vi "VMI_acquire_subV_Arrays.vi"(0 "Big_image Array":i16[][][](array[numeric]), 2 "Queue Array":T7[](array[typedef]), 4 "IMAQ In":T4, 5 "error in (no error)":errorcluster, 7 "Types to acquire in":bool[](array[boolean]), 9 "Collection Information":T1[](array[typedef]), 10 "Peak Find Settings":T6, 11 "Session Out":T3, 13 "Ref Cluster 1":T2) -> (12 "Points per image":i32[](array[numeric]), 14 "IMAQ out":T4, 15 "Histogram_array":i32[][](array[numeric]), 16 "Signal Background":cluster{"X":sgl, "Y":sgl}[](array[cluster]), 17 "Background":cluster{"X":sgl, "Y":sgl}[](array[cluster]), 18 "Background 2":cluster{"X":sgl, "Y":sgl}[](array[cluster]), 19 "error out":errorcluster)   [LabVIEW 2018]
uses:
  <vilib>/vision/Image Controls.llb/IMAQ Image.ctl
  <vilib>/userdefined/High Color/IMAQdx.ctl
  Type defs/Ref_cluster.ctl
  Type defs/FileAcq_v1_Ctrl.ctl
panel:
  out "Graph X":i32[](array[numeric])
  in  "Back2_Points_Image":i32[](array[numeric])
  in  "Back1_Points_Image":i32[](array[numeric])
  in  "Signal_Points_Image":i32[](array[numeric])
  in  "Types to acquire settings":T5(array[cluster])
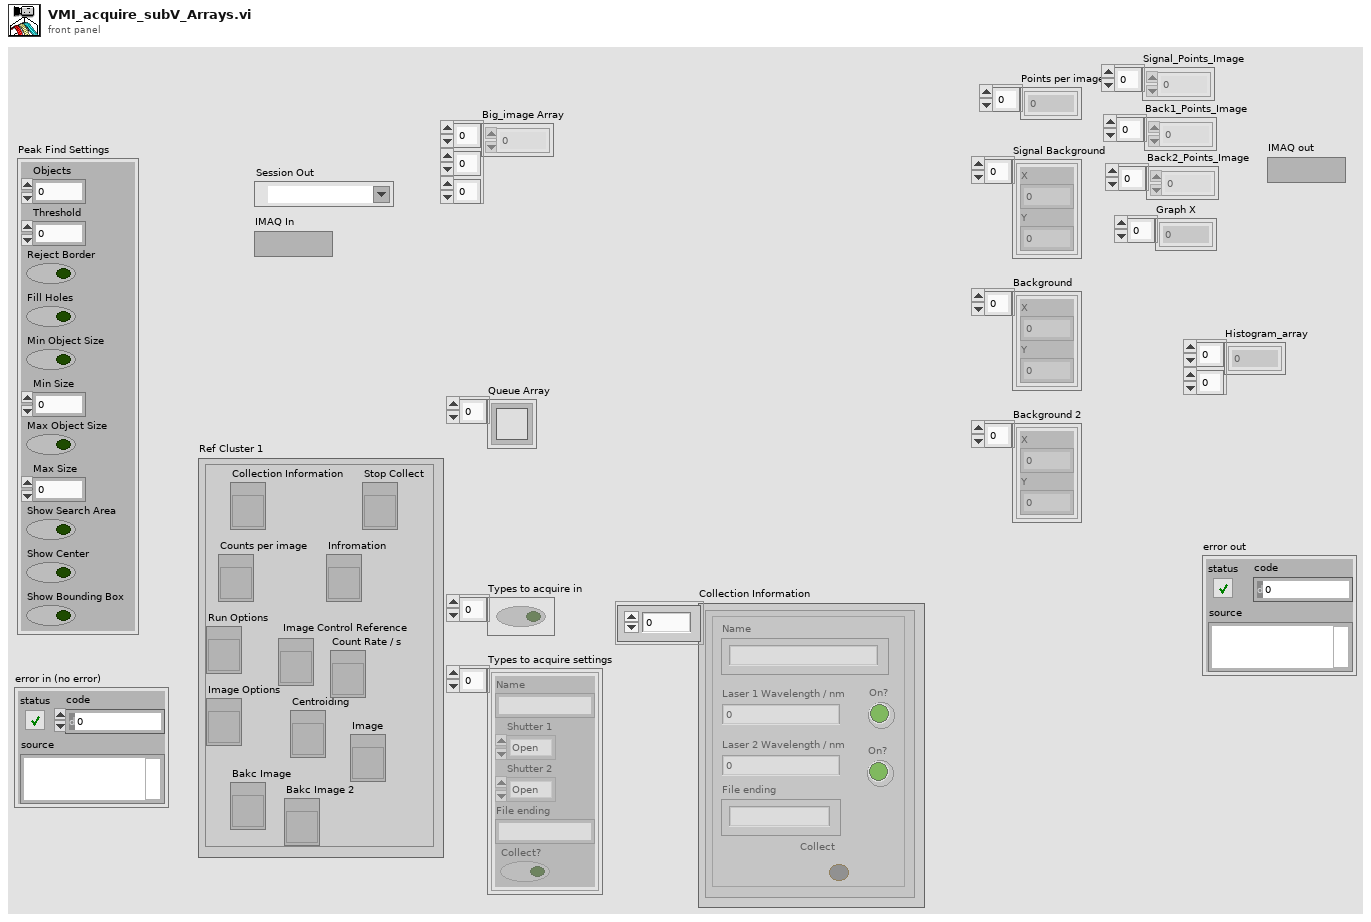
[diagram p1: front panel]
types:
  T1 = typedef "FileAcq_v1_Ctrl.ctl" = cluster{"Type":string, "LaserWave1":dbl, "Shutter1":bool, "LaserWave2":dbl, "Shutter2":bool, "FileEnd":string, "Collect":bool}
  T2 = typedef "Ref_cluster.ctl" = cluster{"Stop Collect ":refnum<vi>, "Collection Information ":refnum<vi>, "Infromation":refnum<vi>, "Counts per image":refnum<vi>, " Image Control Reference ":refnum<vi>, "Run Options":refnum<vi>, "Image Options":refnum<vi>, "Centroiding":refnum<vi>, "Image":refnum<vi>, "Bakc Image":refnum<vi>, "Bakc Image 2":refnum<vi>, "Count Rate / s":refnum<vi>}
  T3 = typedef "IMAQdx.ctl" = refnum<k21>
  T4 = typedef "IMAQ Image.ctl" = refnum<image>
  T5 = cluster{"Name":string, "Shutter 1":enum16{"Open", "Closed"}, "Shutter 2":enum16{"Open", "Closed"}, "File ending":string, "Collect?":bool}[]
  T6 = cluster{"Objects":u16, "Threshold":i32, "Reject Border":bool, "Fill Holes":bool, "Min Object Size":bool, "Min Size":i32, "Max Object Size":bool, "Max Size":i32, "Show Search Area":bool, "Show Center":bool, "Show Bounding Box":bool}
  T7 = typedef "Queue RefNum" = refnum<k1>
  T8 = typedef "Image Type" = u32
  T9 = cluster{"Total Time / ms":dbl, "Image Total Collection Time":dbl, "Image Loop time / ms":dbl, "Peak Total Find Time":dbl, "Peak Find Time / ms":dbl, "Camera Rate / Hz":dbl, "Total Number of Loops":dbl, "Current Loop Number":dbl, "Number of Image Loops":dbl, "Run Mode":dbl}
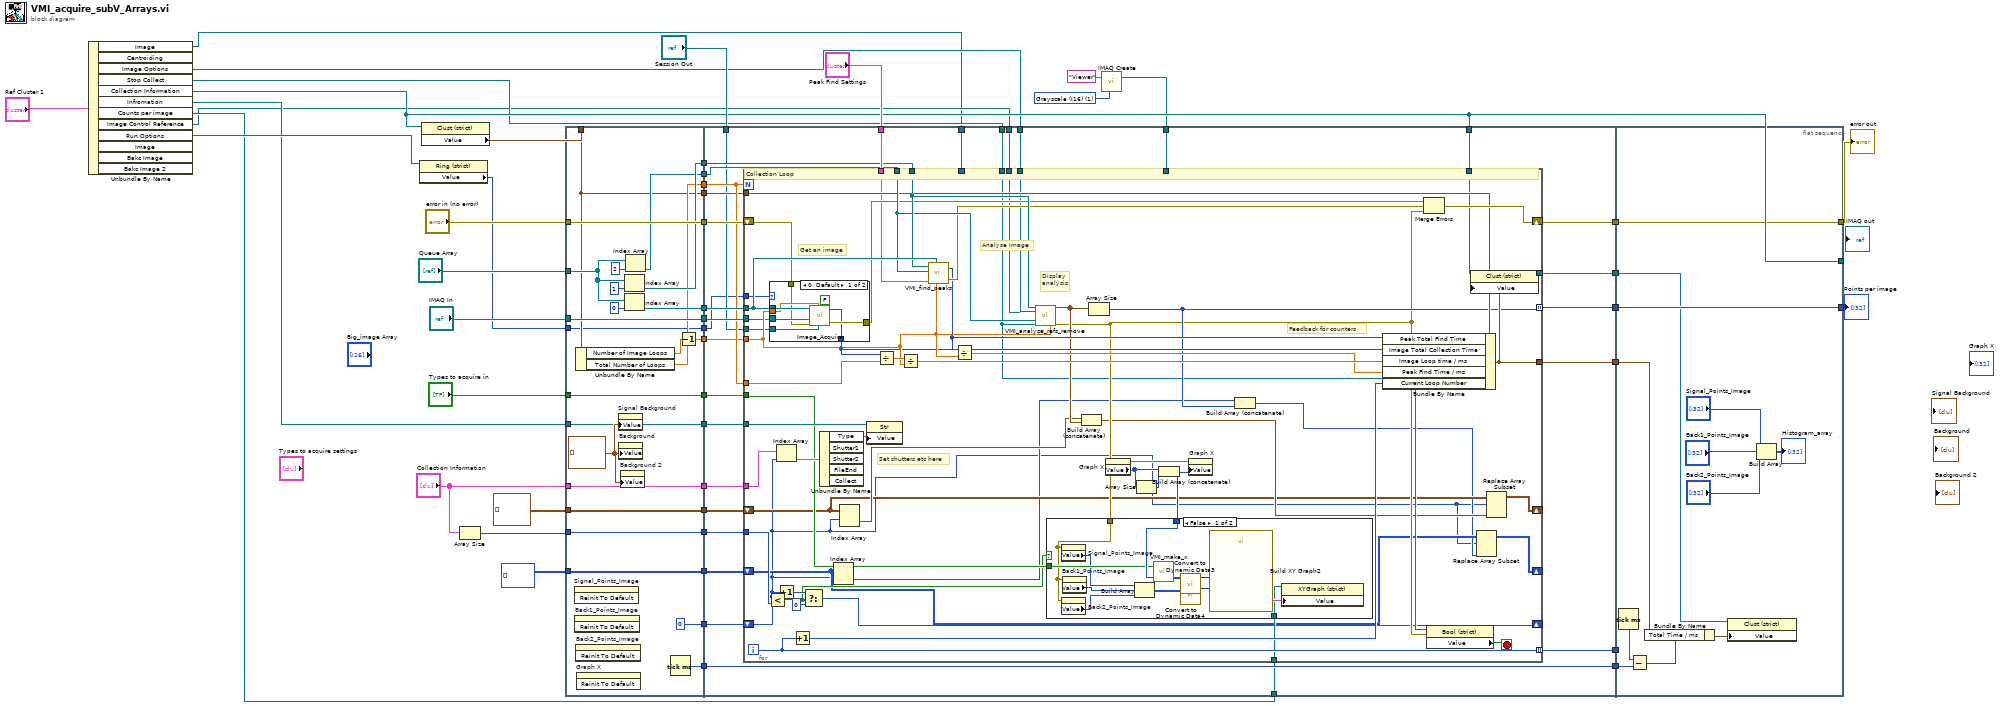
[diagram p0: block diagram]
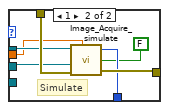
[diagram p2: hidden frame]
diagram:
  w9 = T8 1 items=["Grayscale (U8)", "Grayscale (I16)", "Grayscale (SGL)", "Complex (CSG)", "RGB (U32)", "HSL (U32)", "RGB (U64)", "Grayscale (U16)"] ("Image Type")
  n1 = Unbundle By Name("Ref Cluster 1") -> ("Image"=w12:refnum<vi>, "Image Options"=w13:refnum<vi>, "Stop Collect"=w17:refnum<vi>, "Collection Information"=w19:refnum<vi>, "Infromation"=w15:refnum<vi>, "Counts per image"=w18:refnum<vi>, "Image Control Reference"=w14:refnum<vi>, "Run Options"=w22:refnum<vi>)  [unwired: 4 out]
  n2 = property class="Ring (strict)"(reference=w22) -> ("Value"=w20:u16)  [unwired: 1 in, 2 out]
  n3 = property class="Clust (strict)"(reference=w19) -> ("Value"=w25:T9)  [unwired: 1 in, 2 out]
  n4 = Array Size(array="Collection Information") -> (size(s)=w4:i32)
  n5 = flat-sequence {
    tunnel: "error in (no error)" -> [w70]
    tunnel: "Collection Information" -> [w71]
    tunnel: "IMAQ In" -> [w72]
    tunnel: [w65] -> w49
    tunnel: [w72] -> w48
    tunnel: [w71] -> w47
    tunnel: [w70] -> w46
    tunnel: [w57] -> w45
    tunnel: [w58] -> w44
    tunnel: [w69] -> w43
    tunnel: [0] -> w42
    tunnel: [w68] -> w41
    tunnel: "Types to acquire in" -> [w68]
    tunnel: [w56] -> w40
    tunnel: "Queue Array" -> [w61]
    tunnel: [w63] -> w39
    tunnel: [w60] -> w38
    tunnel: w25 -> [w56]
    tunnel: [w54] -> w21
    tunnel: w20 -> [w54]
    tunnel: [w53] -> w16
    tunnel: w15 -> [w53]
    tunnel: cluster{"X":sgl, "Y":sgl}[][] [] -> [w52]
    tunnel: [w52] -> w6
    tunnel: w4 -> [w51]
    tunnel: [w51] -> w3
    tunnel: [w50] -> w2
    tunnel: i32[][] [] ("Histogram_array 2") -> [w50]
    tunnel: [w102] -> w37
    tunnel: [w99] -> w36
    tunnel: [w98] -> w35
    tunnel: w49 -> [w103]
    tunnel: w48 -> [w101]
    tunnel: w47 -> [w100]
    tunnel: w46 -> [w97]
    tunnel: w45 -> [w96]
    tunnel: w44 -> [w95]
    tunnel: [w94] -> w34
    tunnel: w43 -> [w94]
    tunnel: w42 -> [w93]
    tunnel: w41 -> [w85]
    tunnel: w40 -> [w92]
    tunnel: [w91] -> w33
    tunnel: "Peak Find Settings" -> [w90]
    tunnel: w39 -> [w89]
    tunnel: w38 -> [w88]
    tunnel: w19 -> [w87]
    tunnel: [w86] -> w24
    tunnel: w18 -> [w84]
    tunnel: "Session Out" -> [w83]
    tunnel: w21 -> [w82]
    tunnel: w17 -> [w81]
    tunnel: w16 -> [w80]
    tunnel: w14 -> [w79]
    tunnel: w13 -> [w78]
    tunnel: w12 -> [w77]
    tunnel: w8 -> [w76]
    tunnel: w6 -> [w75]
    tunnel: w3 -> [w74]
    tunnel: w2 -> [w73]
    tunnel: [w196] -> w28
    tunnel: [w197] -> w26
    tunnel: w37 -> [w197]
    tunnel: w36 -> [w196]
    tunnel: w35 -> [_]
    tunnel: w34 -> [w194]
    tunnel: w33 -> [w192]
    tunnel: w19 -> [_]
    tunnel: w24 -> [w190]
    frame #0 {
      w55 = cluster{"X":sgl, "Y":sgl}[] []
      n6 = invoke on="Signal_Points_Image" class="Arr (strict)" method="Reinit To Default"() -> ()  [unwired: 3 in, 3 out]
      n7 = invoke on="Back1_Points_Image" class="Arr (strict)" method="Reinit To Default"() -> ()  [unwired: 3 in, 3 out]
      n8 = Unbundle By Name(w56) -> ("Number of Image Loops"=w59:dbl, "Total Number of Loops"=w57:dbl)
      n9 = invoke on="Back2_Points_Image" class="Arr (strict)" method="Reinit To Default"() -> ()  [unwired: 3 in, 3 out]
      n10 = invoke on="Graph X" class="Arr (strict)" method="Reinit To Default"() -> ()  [unwired: 3 in, 3 out]
      n11 = property on="Signal Background" class="Arr (strict)"("Value"=w55) -> ()  [unwired: 2 in, 2 out]
      n12 = property on="Background" class="Arr (strict)"("Value"=w55) -> ()  [unwired: 2 in, 2 out]
      n13 = property on="Background 2" class="Arr (strict)"("Value"=w55) -> ()  [unwired: 2 in, 2 out]
      n14 = Index Array(array=w61, index=1) -> (element=w63:T7)
      n15 = Index Array(array=w61, index=0) -> (element=w65:T7)
      n16 = Index Array(array=w61, index=2) -> (element=w60:T7)
      n17 = Tick Count (ms)() -> (millisecond timer value=w69:u32)
      n18 = Decrement(x=w59) -> (x-1=w58:dbl)
    }
    frame #1 {
      n19 = for {
        N: w96 -> [_]
        tunnel: w101 -> [w120]
        tunnel: w103 -> [w158]
        tunnel: w89 -> [w157]
        tunnel: w88 -> [w156]
        tunnel: w95 -> [w148]
        shift-right: [w155] -> w102
        shift-left: w97 -> [w124]
        tunnel: w100 -> [w147]
        tunnel: [w132] -> w99 mode=indexing
        tunnel: [w152] -> w98 mode=indexing
        tunnel: w96 -> [w151]
        tunnel: w85 -> [w126]
        shift-right: [w114] -> _
        shift-left: w93 -> [w105]
        tunnel: w92 -> [w146]
        tunnel: [w138] -> w91
        tunnel: w90 -> [w140]
        tunnel: w80 -> [w139]
        tunnel: w87 -> [w137]
        tunnel: [w136] -> w86
        tunnel: w84 -> [w125]
        tunnel: w83 -> [w123]
        tunnel: w82 -> [w122]
        tunnel: w81 -> [w121]
        tunnel: w79 -> [w118]
        tunnel: w78 -> [w119]
        tunnel: w77 -> [_]
        tunnel: w76 -> [_]
        tunnel: w74 -> [w116]
        shift-right: [w109] -> _
        shift-left: w75 -> [w110]
        shift-right: [w104] -> _
        shift-left: w73 -> [w107]
        i -> [w152]
        stop <- w149 stop-if-true
        # "Set shutters etc here"
        # "Feedback for counters"
        # "Display \nanalysis"
        # "Analyse Image"
        # "Get an image"
        # "Collection Loop"
        n20 = Less?(x=w105, y=w116) -> (x < y?=w113:bool)
        n21 = case shown="0, Default" w122 {
          tunnel: w120 -> [w166 w171]
          tunnel: w158 -> [w165 w170]
          tunnel: [w164 w172] -> w154
          tunnel: w148 -> [w162 w167]
          tunnel: [w161 w169] -> w145
          tunnel: w124 -> [w160 w173]
          tunnel: w123 -> [w159 _]
          frame 0, Default {
            n22 = call "Image_Acquire.vi"("Queue Ref in"=w165, "Acquire Time"=w162, "Image Out"=w166, "Session In"=w159, "error in (no error)"=w160, "Test Timing"=FALSE) -> ("Loop Time Out"=w161:i64, "error out"=w164:errorcluster)  [unwired: 1 in]
          }
          frame 1 {
            # "Simulate"
            n23 = call "Image_Acquire_simulate.vi"("Queue Ref in"=w170, "Acquire Time"=w167, "Image Out"=w171, "error in (no error)"=w173, "Test Timing"=FALSE) -> ("Loop Time Out"=w169:i64, "error out"=w172:errorcluster)  [unwired: 2 in]
          }
        }
        n24 = Index Array(array=w147, index=w105) -> (element=w135:T1)
        n25 = Increment(x=w105) -> (x+1=w115:i32)
        n26 = Increment(x=w152) -> (x+1=w142:i32)
        n27 = Select(t=w115, s=w113, f=0) -> (s? t:f=w114:i32)
        n28 = Unbundle By Name(w135) -> ("Type"=w134:string)  [unwired: 4 out]
        n29 = Index Array(array=w107, index (row)=w105) -> (element=w108:i32[])  [unwired: 1 in]
        n30 = Index Array(array=w110, index (row)=w105) -> (element=w112:cluster{"X":sgl, "Y":sgl}[])  [unwired: 1 in]
        n31 = property class="Str"(reference=w139, "Value"=w134) -> ()  [unwired: 1 in, 2 out]
        n32 = Divide(x=w145, y=w151) -> (x/y=w153:dbl)
        n33 = Divide(x=w153, y=w148) -> (x/y=w144:dbl)
        n34 = call "VMI_find_peaks.vi"("Acquire Time"=w148, "Acquire Queue In"=w158, "Peak Find Settings"=w140, "Image Queue in"=w156, "Peak Position Queue in"=w157) -> ("error out"=w150:errorcluster, "x-y"=w141:u32)  [unwired: 1 in]
        n35 = Divide(x=w141, y=w148) -> (x/y=w143:dbl)
        n36 = call "VMI_analyse_refs_remove.vi"("Peak Position Queue in"=w157, "Image Options"=w119, "Image Control Reference"=w118, "Image in"=w156, "Stop Button Ref"=w121, "Acquire Time"=w148) -> ("Peaks Position Out"=w133:cluster{"X":sgl, "Y":sgl}[], "error out"=w128:errorcluster)  [unwired: 5 in, 3 out]
        n37 = Build Array (concatenate)(w112, w133) -> (w111:cluster{"X":sgl, "Y":sgl}[])
        n38 = Array Size(array=w133) -> (size(s)=w132:i32)
        n39 = property on="Graph X" class="Arr (strict)"(error in=w128) -> (error out=w129:errorcluster, "Value"=w131:i32[])  [unwired: 1 in, 1 out]
        n40 = Array Size(array=w131) -> (size(s)=w130:i32)
        n41 = Build Array (concatenate)(w131, w130) -> (w127:i32[])
        n42 = case shown="False" w113 {
          tunnel: w128 -> [w176 _]
          tunnel: w127 -> [w183 _]
          tunnel: w126 -> [w181 _]
          tunnel: w125 -> [w174 _]
          frame False {
            n43 = property on="Signal_Points_Image" class="Arr (strict)"(error in=w176) -> ("Value"=w179:i32[])  [unwired: 1 in, 2 out]
            n44 = property on="Back2_Points_Image" class="Arr (strict)"(error in=w176) -> ("Value"=w177:i32[])  [unwired: 1 in, 2 out]
            n45 = property on="Back1_Points_Image" class="Arr (strict)"(error in=w176) -> ("Value"=w178:i32[])  [unwired: 1 in, 2 out]
            n46 = Build Array(w179, w178, w177) -> (w180:i32[][])
            n47 = call "VMI_make_x.vi"("Graph X"=w183, "Types to acquire in"=w181) -> ("CompiledX"=w182:i32[][])  [unwired: 1 in]
            n48 = call "Convert to Dynamic Data3"("2D Array"=w182) -> ("Dynamic Data Type"=w185:dynamicdata)  [unwired: 3 in]
            n49 = call "Convert to Dynamic Data4"("2D Array"=w180) -> ("Dynamic Data Type"=w184:dynamicdata)  [unwired: 3 in]
            n50 = call "Build XY Graph2"("Y Input"=w184, "X Input"=w185) -> ("XY Graph"=w175:cluster{"X":dbl[], "Y":dbl[]}[])  [unwired: 8 in, 1 out]
            n51 = property on="Property Node" class="XYGraph (strict)"(reference=w174, "Value"=w175) -> ()  [unwired: 1 in, 2 out]
          }
          frame True {
          }
        }
        n52 = property on="Graph X" class="Arr (strict)"(error in=w129, "Value"=w127) -> ()  [unwired: 1 in, 2 out]
        n53 = Build Array (concatenate)(w108, w132) -> (w106:i32[])
        n54 = Bundle By Name(cluster=w146, "Peak Total Find Time"=w141, "Image Total Collection Time"=w145, "Image Loop time / ms"=w144, "Peak Find Time / ms"=w143, "Current Loop Number"=w142) -> (w138:T9)
        n55 = Merge Errors(w154, w150, w128) -> (w155:errorcluster)
        n56 = property on="Property Node" class="Bool (strict)"(reference=w121, error in=w128) -> ("Value"=w149:bool)  [unwired: 2 out]
        n57 = property on="Property Node" class="Clust (strict)"(reference=w137, "Value"=w138) -> (reference out=w136:refnum<vi>)  [unwired: 1 in, 1 out]
        n58 = Replace Array Subset(array=w107, new element=w106, index (row)=w105) -> (w104:i32[][])  [unwired: 1 in]
        n59 = Replace Array Subset(array=w110, new element=w111, index (row)=w105) -> (w109:cluster{"X":sgl, "Y":sgl}[][])  [unwired: 1 in]
      }
    }
    frame #2 {
      n60 = Tick Count (ms)() -> (millisecond timer value=w195:u32)
      n61 = Subtract(x=w195, y=w194) -> (x-y=w193:u32)
      n62 = Bundle By Name(cluster=w192, "Total Time / ms"=w193) -> (w191:T9)
      n63 = property on="Property Node" class="Clust (strict)"(reference=w190, "Value"=w191) -> ()  [unwired: 1 in, 2 out]
      n64 = Build Array("Signal_Points_Image", "Back1_Points_Image", "Back2_Points_Image") -> (→"Histogram_array":i32[][])
    }
  }
  n65 = call "IMAQ Create"("Image Name"="Viewer", "Image Type"=w9) -> ("New Image"=w8:T4)  [unwired: 3 in, 1 out]
  "Points per image" <- w28
  "error out" <- w26
